vi "aitdtView.vi"   [LabVIEW 2013, in "AITDTViews.lvlib"]
uses:
  AITDTViews.lvlib
  CommandFactory/CommandFactory.lvclass
  UserEvents/UserEvents.lvclass
  UserEvents/UserEvents.lvclass/UserEvents.ctl
  Typedefs/CommandSelector.ctl
  Typedefs/StateSelector.ctl
  temperatureSetpointRequestView.vi
  waitTimeView.vi
  Typedefs/AITDTTypedefs.lvlib
  Controller/Controller.lvclass
  ConfigurationThisComponent/ConfigurationThisComponent.lvclass
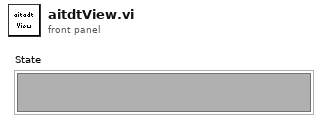
[diagram p1: front panel]
types:
  T1 = enum32{"invalid app kind", "Development System", "Run Time System", "Student Edition", "Embedded LabVIEW", "Evaluation", "Custom"}
  T2 = typedef "AITDTTypedefs.lvlib/PubDataEvents.ctl" = cluster{"State":refnum<user-event>, "ErrorCode":refnum<user-event>, "OutputData":refnum<user-event>, "InputData":refnum<user-event>, "TestStatus":refnum<user-event>, "LogPath":refnum<user-event>, "TemperatureSetpointRequest":refnum<user-event>, "TemperatureSettling":refnum<user-event>, "WaitTimeStatus":refnum<user-event>}
  T3 = typedef "AITDTTypedefs.lvlib/SubDataEvents.ctl" = cluster{"Command":refnum<user-event>}
  T4 = cluster{"Event Registration Refnum":refnum<event-registration>, "Event Registration Refnum":refnum<event-registration>}
  T5 = typedef "AITDTTypedefs.lvlib/CommandSelector.ctl" = enum16{"ClearError", "ConfirmSetpointApplied", "Exit", "StandBy", "Start", "StartTest", "StopTest", "Update"}
  T6 = typedef "AITDTTypedefs.lvlib/StateSelector.ctl" = enum16{"AwaitingSetpointAcknowledgmentState", "EndingCycleState", "FaultState", "OffState", "PausingState", "RequestingNewSetpointState", "SamplingState", "SettlingState", "SoakingState", "StabilizingState", "StandbyState", "StoppedState", "TransitioningTemperatureState"}
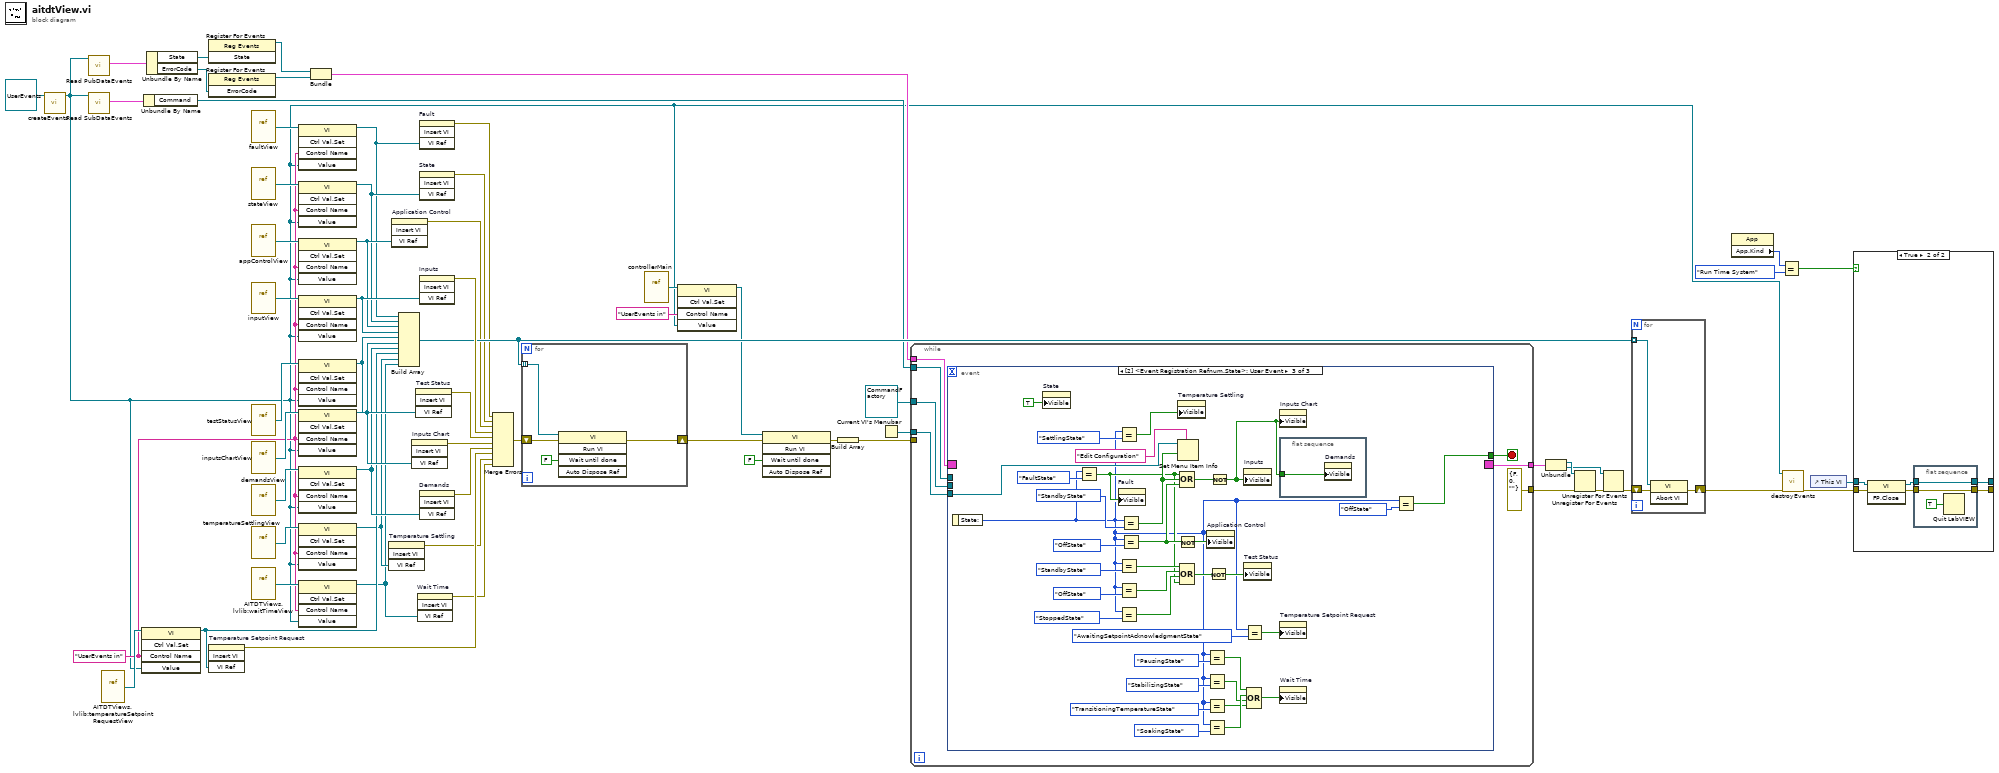
[diagram p0: block diagram]
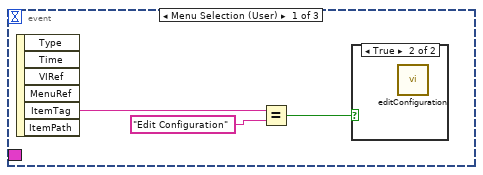
[diagram p3: hidden frame]
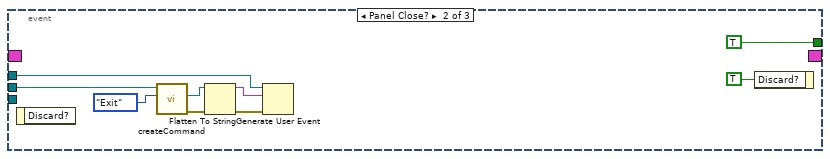
[diagram p5: hidden frame]
diagram:
  w3 = "UserEvents in" ("Control Name")
  n1 = call "createEvents.vi"("UserEvents in"=refnum<class "UserEvents.lvclass"> refnum) -> ("UserEvents out"=w2:refnum<class "UserEvents.lvclass">)  [unwired: 9 in, 1 out]
  n2 = call "Read PubDataEvents.vi"("UserEvents in"=w2) -> ("PubDataEvents"=w56:T2)  [unwired: 9 in, 1 out]
  n3 = call "Read SubDataEvents.vi"("UserEvents in"=w2) -> ("SubDataEvents"=w54:T3)  [unwired: 9 in, 1 out]
  n4 = vi-ref "AITDTViews.lvlib:temperatureSetpointRequestView.vi"() -> (w12:refnum<vi>)
  n5 = invoke class="VI" method="Ctrl Val.Set"(reference=w12, "Control Name"=w3, "Value"=w2) -> (reference out=w10:refnum<vi>)  [unwired: 2 in, 4 out]
  n6 = Unbundle By Name(w54) -> ("Command"=w53:refnum<user-event>)
  n7 = Unbundle By Name(w56) -> ("State"=w52:refnum<user-event>, "ErrorCode"=w50:refnum<user-event>)
  n8 = register-events(w52) -> (reference out=w51:refnum<event-registration>)  [unwired: 2 in, 1 out]
  n9 = register-events(w50) -> (reference out=w49:refnum<event-registration>)  [unwired: 2 in, 1 out]
  n10 = invoke on="Temperature Setpoint Request" class="SubPnl" method="Insert VI"("VI Ref"=w10) -> (error out=w9:errorcluster)  [unwired: 3 in, 3 out]
  n11 = vi-ref "faultView.vi"() -> (w19:refnum<vi>)
  n12 = vi-ref "stateView.vi"() -> (w22:refnum<vi>)
  n13 = vi-ref "appControlView.vi"() -> (w26:refnum<vi>)
  n14 = vi-ref "inputView.vi"() -> (w44:refnum<vi>)
  n15 = vi-ref "testStatusView.vi"() -> (w32:refnum<vi>)
  n16 = vi-ref "inputsChartView.vi"() -> (w29:refnum<vi>)
  n17 = vi-ref "demandsView.vi"() -> (w14:refnum<vi>)
  n18 = vi-ref "temperatureSettlingView.vi"() -> (w8:refnum<vi>)
  n19 = vi-ref "AITDTViews.lvlib:waitTimeView.vi"() -> (w5:refnum<vi>)
  n20 = invoke class="VI" method="Ctrl Val.Set"(reference=w19, "Control Name"=w3, "Value"=w2) -> (reference out=w18:refnum<vi>)  [unwired: 2 in, 4 out]
  n21 = invoke class="VI" method="Ctrl Val.Set"(reference=w22, "Control Name"=w3, "Value"=w2) -> (reference out=w21:refnum<vi>)  [unwired: 2 in, 4 out]
  n22 = invoke class="VI" method="Ctrl Val.Set"(reference=w26, "Control Name"=w3, "Value"=w2) -> (reference out=w24:refnum<vi>)  [unwired: 2 in, 4 out]
  n23 = invoke class="VI" method="Ctrl Val.Set"(reference=w44, "Control Name"=w3, "Value"=w2) -> (reference out=w36:refnum<vi>)  [unwired: 2 in, 4 out]
  n24 = invoke class="VI" method="Ctrl Val.Set"(reference=w32, "Control Name"=w3, "Value"=w2) -> (reference out=w31:refnum<vi>)  [unwired: 2 in, 4 out]
  n25 = invoke class="VI" method="Ctrl Val.Set"(reference=w29, "Control Name"=w3, "Value"=w2) -> (reference out=w27:refnum<vi>)  [unwired: 2 in, 4 out]
  n26 = invoke class="VI" method="Ctrl Val.Set"(reference=w14, "Control Name"=w3, "Value"=w2) -> (reference out=w11:refnum<vi>)  [unwired: 2 in, 4 out]
  n27 = invoke class="VI" method="Ctrl Val.Set"(reference=w8, "Control Name"=w3, "Value"=w2) -> (reference out=w7:refnum<vi>)  [unwired: 2 in, 4 out]
  n28 = invoke class="VI" method="Ctrl Val.Set"(reference=w5, "Control Name"=w3, "Value"=w2) -> (reference out=w1:refnum<vi>)  [unwired: 2 in, 4 out]
  n29 = Bundle("Event Registration Refnum"=w51, "Event Registration Refnum"=w49) -> (w42:T4)  [unwired: 1 in]
  n30 = invoke on="Temperature Settling" class="SubPnl" method="Insert VI"("VI Ref"=w7) -> (error out=w6:errorcluster)  [unwired: 3 in, 3 out]
  n31 = invoke on="Application Control" class="SubPnl" method="Insert VI"("VI Ref"=w24) -> (error out=w25:errorcluster)  [unwired: 3 in, 3 out]
  n32 = Build Array(w18, w21, w24, w36, w31, w27, w11, w10, w7, w1) -> (w59:refnum<vi>[])
  n33 = invoke on="Inputs Chart" class="SubPnl" method="Insert VI"("VI Ref"=w27) -> (error out=w28:errorcluster)  [unwired: 3 in, 3 out]
  n34 = invoke on="Test Status" class="SubPnl" method="Insert VI"("VI Ref"=w31) -> (error out=w30:errorcluster)  [unwired: 3 in, 3 out]
  n35 = invoke on="Wait Time" class="SubPnl" method="Insert VI"("VI Ref"=w1) -> (error out=w4:errorcluster)  [unwired: 3 in, 3 out]
  n36 = invoke on="Fault" class="SubPnl" method="Insert VI"("VI Ref"=w18) -> (error out=w17:errorcluster)  [unwired: 3 in, 3 out]
  n37 = invoke on="State" class="SubPnl" method="Insert VI"("VI Ref"=w21) -> (error out=w20:errorcluster)  [unwired: 3 in, 3 out]
  n38 = invoke on="Inputs" class="SubPnl" method="Insert VI"("VI Ref"=w36) -> (error out=w61:errorcluster)  [unwired: 3 in, 3 out]
  n39 = invoke on="Demands" class="SubPnl" method="Insert VI"("VI Ref"=w11) -> (error out=w13:errorcluster)  [unwired: 3 in, 3 out]
  n40 = Merge Errors(w17, w20, w25, w61, w30, w28, w13, w9, w6, w4) -> (w60:errorcluster)
  n41 = for {
    tunnel: w59 -> [w68] mode=indexing
    shift-right: [w67] -> w23
    shift-left: w60 -> [w66]
    n42 = invoke class="VI" method="Run VI"(reference=w68, error in=w66, "Wait until done"=FALSE ("Wait Until Done")) -> (error out=w67:errorcluster)  [unwired: 2 in, 4 out]
  }
  n43 = vi-ref "controllerMain.vi"() -> (w47:refnum<vi>)
  n44 = invoke class="VI" method="Ctrl Val.Set"(reference=w47, "Control Name"="UserEvents in", "Value"=w2) -> (reference out=w45:refnum<vi>)  [unwired: 2 in, 4 out]
  n45 = invoke class="VI" method="Run VI"(reference=w45, error in=w23, "Wait until done"=FALSE ("Wait Until Done")) -> (error out=w33:errorcluster)  [unwired: 2 in, 4 out]
  n46 = Build Array(w33) -> (w34:errorcluster[])
  n47 = Current VI's Menubar() -> (w57:refnum<k9>)
  n48 = while {
    tunnel: refnum<class "CommandFactory.lvclass"> refnum ("CommandFactory.lvclass") -> [w72]
    tunnel: [errorcluster {"status"=FALSE, "code"=0, "source"=""} ("error out")] -> w43
    tunnel: w57 -> [w70]
    tunnel: w42 -> [w74]
    tunnel: w53 -> [w71]
    tunnel: [w69] -> w41
    tunnel: w34 -> [_]
    stop <- w73 stop-if-true
    n49 = event shown="[2] <Event Registration Refnum.State>: User Event" {
      selector: w74 -> [_ _ _]
      dyn-events: [_ _ _] -> w69
      timeout: _ -> [_ _ _]
      tunnel: [_ TRUE w117] -> w73
      tunnel: w72 -> [_ w82 _]
      tunnel: w71 -> [_ w79 _]
      tunnel: w70 -> [_ _ w119]
      event Menu Selection (User) {
        n50 = event-data() -> ("ItemTag"=w76:string)  [unwired: 1 in, 5 out]
        n51 = Equal?(x=w76, y="Edit Configuration") -> (x = y?=w78:bool)
        n52 = case shown="True" w78 {
          frame False {
          }
          frame True {
            n53 = call "editConfiguration.vi"() -> ()  [unwired: 10 in, 2 out]
          }
        }
      }
      event Panel Close? {
        n54 = event-data() -> ()  [unwired: 1 in, 1 out]
        n55 = call-dynamic "createCommand.vi"("Command"=CommandSelector."Exit", "CommandFactory in"=w82) -> ("error out"=w87:errorcluster, "command"=w86:refnum<class "Command.lvclass">)  [unwired: 7 in, 1 out]
        n56 = Flatten To String(anything=w86, error in (no error)=w87) -> (data string=w80:string, error out=w81:errorcluster)  [unwired: 2 in, 1 out]
        n57 = Generate User Event(user event=w79, event data cluster=w80, error in=w81) -> ()  [unwired: 1 in, 2 out]
        n58 = event-data("Discard?"=TRUE) -> ()  [unwired: 1 in, 1 out]
      }
      event User Event {
        n59 = event-data() -> ("State:"=w88:T6)  [unwired: 1 in]
        n60 = property on="State" class="SubPnl"("Visible"=TRUE) -> ()  [unwired: 2 in, 2 out]
        n61 = Equal?(x=w88, y=StateSelector."FaultState") -> (x = y?=w98:bool)
        n62 = property on="Fault" class="SubPnl"("Visible"=w98) -> ()  [unwired: 2 in, 2 out]
        n63 = Equal?(x=w88, y=StateSelector."SettlingState") -> (x = y?=w99:bool)
        n64 = Equal?(x=w88, y=StateSelector."StandbyState") -> (x = y?=w112:bool)
        n65 = Equal?(x=w88, y=StateSelector."OffState") -> (x = y?=w111:bool)
        n66 = Equal?(x=w88, y=StateSelector."StoppedState") -> (x = y?=w101:bool)
        n67 = Equal?(x=w88, y=StateSelector."StandbyState") -> (x = y?=w116:bool)
        n68 = Equal?(x=w88, y=StateSelector."OffState") -> (x = y?=w108:bool)
        n69 = Not(x=w108) -> (.not. x?=w109:bool)
        n70 = property on="Temperature Settling" class="SubPnl"("Visible"=w99) -> ()  [unwired: 2 in, 2 out]
        n71 = Set Menu Item Info(7:"Edit Configuration" ("item name"), 9:w116, 11:w119) -> ()  [unwired: 4 in, 2 out]
        n72 = Compound Arithmetic op=OR(w98, w116, w108) -> (w115:bool)
        n73 = Compound Arithmetic op=OR(w112, w111, w101, w98) -> (w110:bool)
        n74 = property on="Application Control" class="SubPnl"("Visible"=w109) -> ()  [unwired: 2 in, 2 out]
        n75 = Equal?(x=w88, y=StateSelector."PausingState") -> (x = y?=w92:bool)
        n76 = Equal?(x=w88, y=StateSelector."StabilizingState") -> (x = y?=w90:bool)
        n77 = Equal?(x=w88, y=StateSelector."TransitioningTemperatureState") -> (x = y?=w89:bool)
        n78 = Equal?(x=w88, y=StateSelector."SoakingState") -> (x = y?=w91:bool)
        n79 = Not(x=w110) -> (.not. x?=w103:bool)
        n80 = Not(x=w115) -> (.not. x?=w106:bool)
        n81 = property on="Inputs" class="SubPnl"("Visible"=w106) -> ()  [unwired: 2 in, 2 out]
        n82 = property on="Test Status" class="SubPnl"("Visible"=w103) -> ()  [unwired: 2 in, 2 out]
        n83 = Equal?(x=w88, y=StateSelector."AwaitingSetpointAcknowledgmentState") -> (x = y?=w104:bool)
        n84 = Compound Arithmetic op=OR(w92, w91, w90, w89) -> (w96:bool)
        n85 = property on="Inputs Chart" class="SubPnl"("Visible"=w106) -> ()  [unwired: 2 in, 2 out]
        n86 = flat-sequence {
          tunnel: w106 -> [w124]
          frame #0 {
            n87 = property on="Demands" class="SubPnl"("Visible"=w124) -> ()  [unwired: 2 in, 2 out]
          }
        }
        n88 = property on="Temperature Setpoint Request" class="SubPnl"("Visible"=w104) -> ()  [unwired: 2 in, 2 out]
        n89 = property on="Wait Time" class="SubPnl"("Visible"=w96) -> ()  [unwired: 2 in, 2 out]
        n90 = Equal?(x=w88, y=StateSelector."OffState") -> (x = y?=w117:bool)
      }
    }
  }
  n91 = Unbundle(w41) -> ("Event Registration Refnum"=w40:refnum<event-registration>, "Event Registration Refnum"=w38:refnum<event-registration>)
  n92 = Unregister For Events(event registration refnum=w40, error in=w43) -> (error out=w39:errorcluster)
  n93 = Unregister For Events(event registration refnum=w38, error in=w39) -> (error out=w37:errorcluster)
  n94 = for {
    tunnel: w59 -> [w127] mode=indexing
    shift-right: [w125] -> w35
    shift-left: w37 -> [w126]
    n95 = invoke class="VI" method="Abort VI"(reference=w127, error in=w126) -> (error out=w125:errorcluster)  [unwired: 1 in, 2 out]
  }
  n96 = property class="App"() -> ("App.Kind"=w64:T1)  [unwired: 2 in, 2 out]
  n97 = Equal?(x=w64, y=T1."Run Time System") -> (x = y?=w62:bool)
  n98 = call "destroyEvents.vi"("error in (no error)"=w35, "UserEvents in"=w2) -> ("error out"=w15:errorcluster)  [unwired: 8 in, 1 out]
  n99 = control-ref of="This VI"() -> (w16:refnum<vi>)
  n100 = case shown="True" w62 {
    tunnel: w16 -> [w129 w135]
    tunnel: w15 -> [w128 w134]
    tunnel: [w129 w132] -> _
    tunnel: [w128 w130] -> _
    frame False {
    }
    frame True {
      n101 = invoke class="VI" method="FP.Close"(reference=w135, error in=w134) -> (reference out=w131:refnum<vi>, error out=w133:errorcluster)  [unwired: 1 in, 1 out]
      n102 = flat-sequence {
        tunnel: w133 -> [w136]
        tunnel: [w137] -> w132
        tunnel: w131 -> [w137]
        tunnel: [w136] -> w130
        frame #0 {
          n103 = Quit LabVIEW(quit? (T)=TRUE) -> ()
        }
      }
    }
  }
